vi "Set_field.vi"() -> ()   [LabVIEW 2016]
panel:
  in  "Y-Axis Communications Config":T1={"GPIB address"=22, "GPIB bus"=1, "connection ID"=refnum, "IP"="192.168.0.106", "Active Comm Interface"=0, "Serial Port"="", "Programmer Type"=0} {"Programmer Type" items=["Model 430", "Model 420"]; "Active Comm Interface" items=["TCP/IP (Model 430 Only)", "RS232", "IEEE488"]}
  in  "Z-Axis Communications Config":T1={"GPIB address"=22, "GPIB bus"=1, "connection ID"=refnum, "IP"="192.168.0.106", "Active Comm Interface"=0, "Serial Port"="", "Programmer Type"=0} {"Programmer Type" items=["Model 430", "Model 420"]; "Active Comm Interface" items=["TCP/IP (Model 430 Only)", "RS232", "IEEE488"]}
  in  "error in":T2
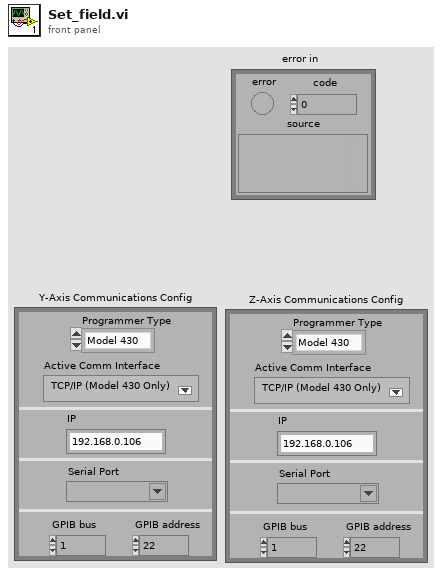
[diagram p1: front panel]
types:
  T1 = cluster{"GPIB address":i16, "GPIB bus":i16, "connection ID":refnum<k5>, "IP":string, "Active Comm Interface":u16, "Serial Port":refnum<visa-resource-name>, "Programmer Type":u16}
  T2 = cluster{"error":bool, "code":i32, "source":string}
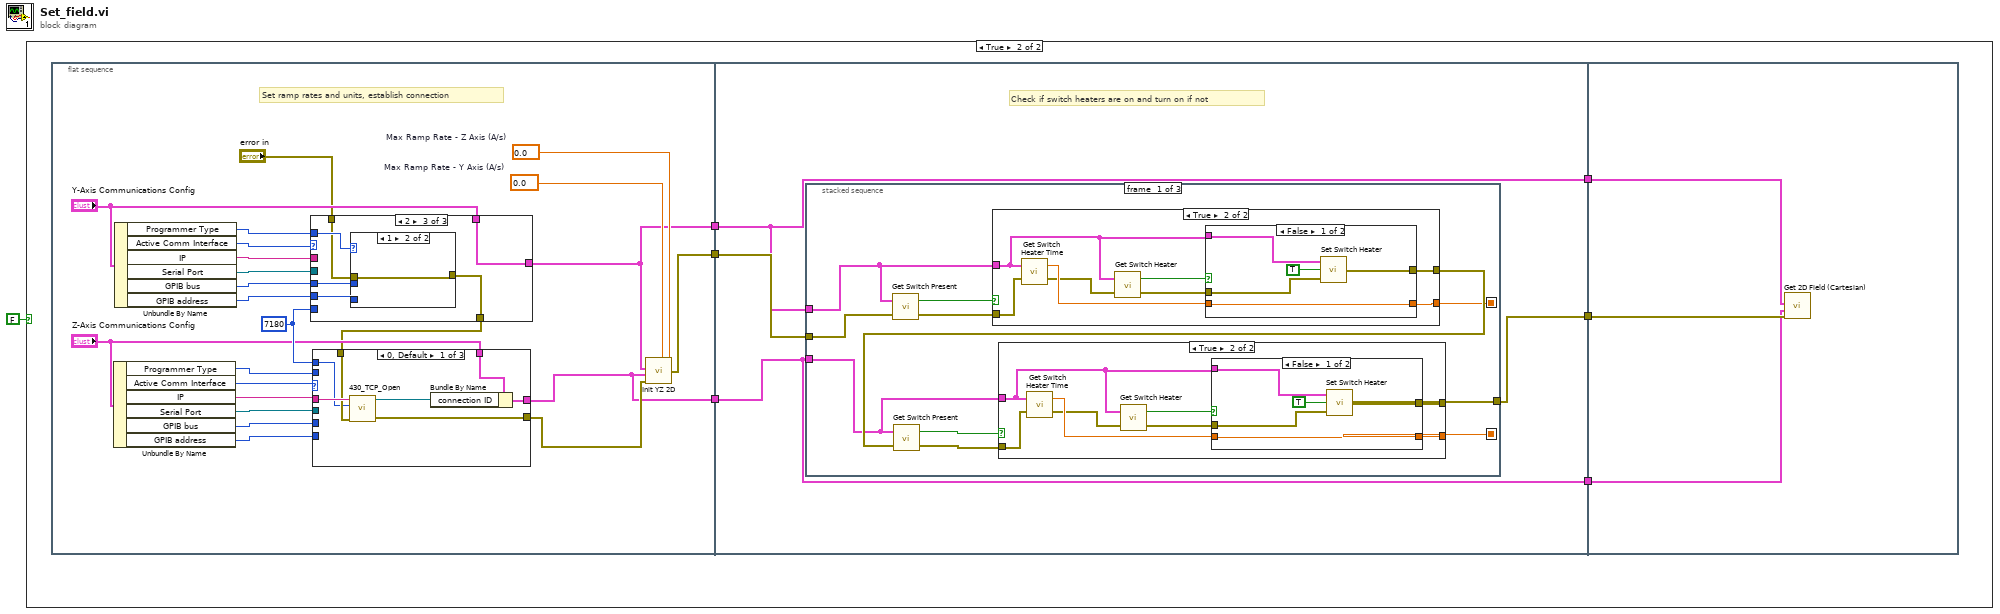
[diagram p0: block diagram]
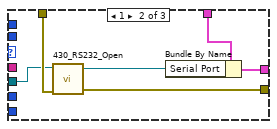
[diagram p3: hidden frame]
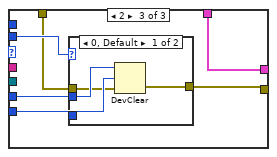
[diagram p4: hidden frame]
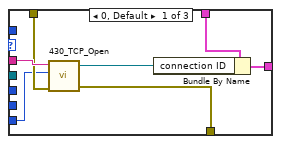
[diagram p6: hidden frame]
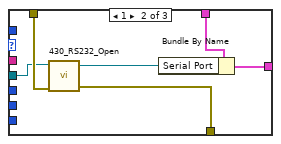
[diagram p7: hidden frame]
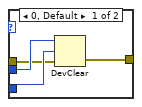
[diagram p8: hidden frame]
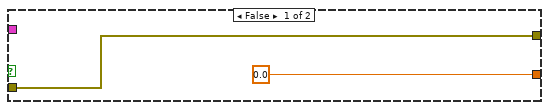
[diagram p9: hidden frame]
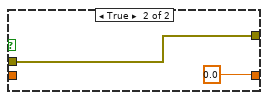
[diagram p10: hidden frame]
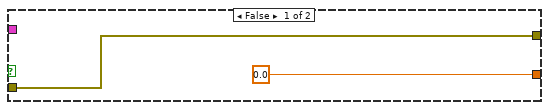
[diagram p11: hidden frame]
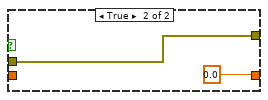
[diagram p12: hidden frame]
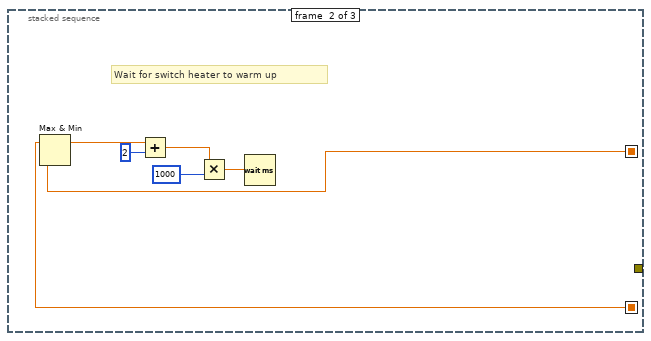
[diagram p13: hidden frame]
diagram:
  n1 = case shown="True" FALSE {
    frame False {
    }
    frame True {
      n2 = flat-sequence {
        tunnel: [w10] -> w7
        tunnel: [w9] -> w6
        tunnel: [w8] -> w5
        tunnel: w7 -> [w81]
        tunnel: w6 -> [w79]
        tunnel: w5 -> [w82]
        tunnel: [w81] -> w4
        tunnel: [w80] -> w3
        tunnel: [w79] -> w2
        tunnel: w4 -> [w137]
        tunnel: w3 -> [w136]
        tunnel: w2 -> [w135]
        frame #0 {
          w12 = 0.0  # Max Ramp Rate - Y Axis (A/s)
          w11 = 0.0  # Max Ramp Rate - Z Axis (A/s)
          w30 = 7180 ("TCP Port")
          # "Set ramp rates and units, establish connection"
          n3 = Unbundle By Name("Z-Axis Communications Config") -> ("Programmer Type"=w21:u16, "Active Comm Interface"=w29:u16, "IP"=w26:string, "Serial Port"=w25:refnum<visa-resource-name>, "GPIB bus"=w20:i16, "GPIB address"=w19:i16)
          n4 = Unbundle By Name("Y-Axis Communications Config") -> ("Programmer Type"=w15:u16, "Active Comm Interface"=w28:u16, "IP"=w27:string, "Serial Port"=w24:refnum<visa-resource-name>, "GPIB bus"=w16:i16, "GPIB address"=w17:i16)
          n5 = case shown="2" w28 {
            tunnel: w27 -> [w61 _ _]
            tunnel: "error in" -> [w60 w67 w69]
            tunnel: "Y-Axis Communications Config" -> [w59 w62 w73]
            tunnel: [w57 w65 w73] -> w10
            tunnel: [w56 w66 w68] -> w18
            tunnel: w30 -> [w55 _ _]
            tunnel: w24 -> [_ w63 _]
            tunnel: w17 -> [_ _ w72]
            tunnel: w16 -> [_ _ w71]
            tunnel: w15 -> [_ _ w70]
            frame 0, Default {
              n6 = call "430_TCP_Open.vi"("IP Address"=w61, "TCP Port"=w55, "error in (no error)"=w60) -> ("connection ID"=w58:refnum<k5>, "error out"=w56:errorcluster)  [unwired: 3 in, 1 out]
              n7 = Bundle By Name(cluster=w59, "connection ID"=w58) -> (w57:T1)
            }
            frame 1 {
              n8 = call "430_RS232_Open.vi"("VISA resource name"=w63, "error in (no error)"=w67) -> ("VISA resource name out"=w64:refnum<visa-resource-name>, "error out"=w66:errorcluster)  [unwired: 5 in]
              n9 = Bundle By Name(cluster=w62, "Serial Port"=w64) -> (w65:T1)
            }
            frame 2 {
              n10 = case shown="1" w70 {
                tunnel: w71 -> [w77 _]
                tunnel: w72 -> [w76 _]
                tunnel: w69 -> [w75 w78]
                tunnel: [w74 w78] -> w68
                frame 0, Default {
                  n11 = DevClear(2:w75, 3:w76, 4:w77) -> (0:w74:errorcluster)  [unwired: 1 out]
                }
                frame 1 {
                }
              }
            }
          }
          n12 = case shown="0, Default" w29 {
            tunnel: w26 -> [w37 _ _]
            tunnel: w18 -> [w36 w43 w45]
            tunnel: [w35 w42 w44] -> w13
            tunnel: "Z-Axis Communications Config" -> [w34 w40 w49]
            tunnel: [w32 w41 w49] -> w9
            tunnel: w30 -> [w31 _ _]
            tunnel: w25 -> [_ w38 _]
            tunnel: w21 -> [_ _ w48]
            tunnel: w20 -> [_ _ w47]
            tunnel: w19 -> [_ _ w46]
            frame 0, Default {
              n13 = call "430_TCP_Open.vi"("IP Address"=w37, "TCP Port"=w31, "error in (no error)"=w36) -> ("connection ID"=w33:refnum<k5>, "error out"=w35:errorcluster)  [unwired: 3 in, 1 out]
              n14 = Bundle By Name(cluster=w34, "connection ID"=w33) -> (w32:T1)
            }
            frame 1 {
              n15 = call "430_RS232_Open.vi"("VISA resource name"=w38, "error in (no error)"=w43) -> ("VISA resource name out"=w39:refnum<visa-resource-name>, "error out"=w42:errorcluster)  [unwired: 5 in]
              n16 = Bundle By Name(cluster=w40, "Serial Port"=w39) -> (w41:T1)
            }
            frame 2 {
              n17 = case shown="0, Default" w48 {
                tunnel: w47 -> [w53 _]
                tunnel: w46 -> [w52 _]
                tunnel: w45 -> [w51 w54]
                tunnel: [w50 w54] -> w44
                frame 0, Default {
                  n18 = DevClear(2:w51, 3:w52, 4:w53) -> (0:w50:errorcluster)  [unwired: 1 out]
                }
                frame 1 {
                }
              }
            }
          }
          n19 = call "Init YZ 2D.vi"("Max Ramp Rate Z-axis"=w11, "Max Ramp Rate Y-axis"=w12, "error in"=w13, "Z-Axis Communications Config"=w9, "Y-Axis Communications Config"=w10) -> ("error out"=w8:T2)  [unwired: 5 in]
        }
        frame #1 {
          # "Check if switch heaters are on and turn on if not"
          n20 = stacked-sequence {
            seq-local: [w85 _ _] -> [_ w129 _]
            seq-local: [w84 _ _] -> [_ w128 _]
            tunnel: w79 -> [w87 _ _]
            tunnel: w82 -> [w88 _ _]
            tunnel: [w83 _ _] -> w80
            tunnel: w81 -> [w86 _ _]
            frame #0 {
              n21 = call "Get Switch Present.vi"("error in"=w88, "Communications Config"=w86) -> ("error out"=w92:T2, "Switch Present?"=w93:bool)
              n22 = case shown="True" w93 {
                tunnel: w92 -> [w111 w120]
                tunnel: w86 -> [_ w113]
                tunnel: [0.0 w117] -> w84
                tunnel: [w111 w119] -> w91
                frame False {
                }
                frame True {
                  n23 = call "Get Switch Heater Time.vi"("error in"=w120, "Communications Config"=w113) -> ("error out"=w116:T2, "Switch Heating Time (secs)"=w118:dbl)
                  n24 = call "Get Switch Heater.vi"("error in"=w116, "Communications Config"=w113) -> ("error out"=w115:T2, "Switch Heater Indicator"=w114:bool)
                  n25 = case shown="False" w114 {
                    tunnel: [w125 w126] -> w119
                    tunnel: w118 -> [w123 _]
                    tunnel: [w123 0.0] -> w117
                    tunnel: w115 -> [w121 w126]
                    tunnel: w113 -> [w122 _]
                    frame False {
                      n26 = call "Set Switch Heater.vi"("error in"=w121, "Switch Heater Control"=TRUE, "Communications Config"=w122) -> ("error out"=w125:T2)
                    }
                    frame True {
                    }
                  }
                }
              }
              n27 = call "Get Switch Present.vi"("error in"=w91, "Communications Config"=w87) -> ("error out"=w89:T2, "Switch Present?"=w90:bool)
              n28 = case shown="True" w90 {
                tunnel: w89 -> [w94 w103]
                tunnel: w87 -> [_ w96]
                tunnel: [0.0 w100] -> w85
                tunnel: [w94 w102] -> w83
                frame False {
                }
                frame True {
                  n29 = call "Get Switch Heater Time.vi"("error in"=w103, "Communications Config"=w96) -> ("error out"=w99:T2, "Switch Heating Time (secs)"=w101:dbl)
                  n30 = call "Get Switch Heater.vi"("error in"=w99, "Communications Config"=w96) -> ("error out"=w98:T2, "Switch Heater Indicator"=w97:bool)
                  n31 = case shown="False" w97 {
                    tunnel: [w104 w109] -> w102
                    tunnel: w101 -> [w107 _]
                    tunnel: [w107 0.0] -> w100
                    tunnel: w98 -> [w105 w109]
                    tunnel: w96 -> [w106 _]
                    frame False {
                      n32 = call "Set Switch Heater.vi"("error in"=w105, "Switch Heater Control"=TRUE, "Communications Config"=w106) -> ("error out"=w104:T2)
                    }
                    frame True {
                    }
                  }
                }
              }
            }
            frame #1 {
              # "Wait for switch heater to warm up"
              n33 = Max & Min(x=w129, y=w128) -> (max(x,y)=w130:dbl)  [unwired: 1 out]
              n34 = Add(x=w130, y=2) -> (x+y=w132:dbl)
              n35 = Multiply(x=w132, y=1000) -> (x*y=w131:dbl)
              n36 = Wait (ms)(milliseconds to wait=w131) -> ()  [unwired: 1 out]
            }
            frame #2 {
            }
          }
        }
        frame #2 {
          n37 = call "Get 2D Field (Cartesian).vi"("Y-Axis Communications Config"=w137, "Z-Axis Communications Config"=w135, "error in"=w136) -> ()  [unwired: 2 in, 4 out]
        }
      }
    }
  }
